vi "Add To DAQmx Task.vi"(6 "Ignore Cal? (F)":bool, 7 "Thermocouple in":refnum<class "Thermocouple.lvclass">, 8 "error in (no error)":errorcluster, 9 "Scale Name":string, 10 "Chassis Name":string, 11 "task in":refnum<k21>) -> (0 "error out":errorcluster, 2 "Phys Chan Added":string, 3 "task out":refnum<k21>)   [LabVIEW 2018, in "Measurement Channels.lvlib" / "Thermocouple.lvclass"]
uses:
  Thermocouple.lvclass
  C:/Users/Jeff Tipps/Documents/DAQMan/source/Classes/Measurements/Class Channel/Channel.lvclass
  Thermocouple.lvclass/Thermocouple.ctl
  Class Channel/Read ChanName.vi
  Class Channel/Read Alias.vi
  <vilib>/DAQmx/create/channels.llb/DAQmx Create Channel (AI-Temperature-Thermocouple).vi
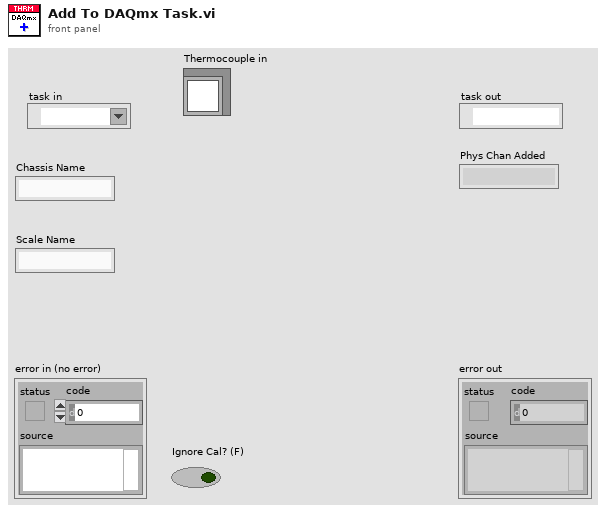
[diagram p1: front panel]
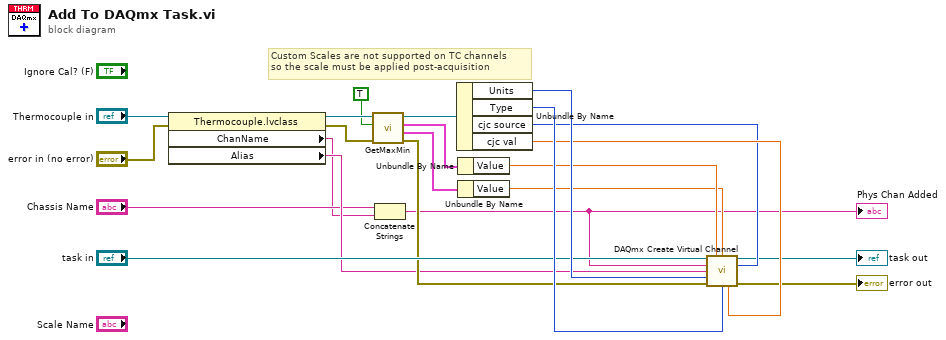
[diagram p0: block diagram]
diagram:
  # "Custom Scales are not supported on TC channels\nso the scale must be applied post-acquisition"
  n1 = property class="Thermocouple.lvclass"(reference="Thermocouple in", error in="error in (no error)") -> (reference out=w13:refnum<class "Thermocouple.lvclass">, error out=w10:errorcluster, "ChanName"=w7:string, "Alias"=w9:string)
  n2 = call-dynamic "GetMaxMin.vi"("error in (no error)"=w10, "Ignore Cal? (F)"=TRUE, "Thermocouple in"=w13) -> ("error out"=w11:errorcluster, "Min"=w5:cluster{"Value":dbl, "Text":string}, "Max"=w6:cluster{"Value":dbl, "Text":string}, "Thermocouple out"=w12:refnum<class "Thermocouple.lvclass">)  [unwired: 5 in]
  n3 = Concatenate Strings("Chassis Name", w7) -> (w2:string)
  "Phys Chan Added" <- w2
  n4 = Unbundle By Name(w12) -> ("Units"=w21:u16, "Type"=w22:u16, "cjc source"=w19:u16, "cjc val"=w20:dbl)
  n5 = Unbundle By Name(w6) -> ("Value"=w4:dbl)
  n6 = Unbundle By Name(w5) -> ("Value"=w3:dbl)
  n7 = call-poly <vilib>:"DAQmx Create Virtual Channel.vi"("task in"="task in", "maximum value"=w4, "minimum value"=w3, "physical channels"=w2, "cjc source"=w19, "name to assign"=w9, "units"=w21, "error in"=w11, "thermocouple type"=w22, "cjc value"=w20) -> ("task out"=→"task out":refnum<k21>, "error out"=→"error out":errorcluster)  [unwired: 4 in]
